vi "Analysis.SingleChannelLevelTransitionLogic.vi"(9 "Stimulus":dbl[](array[numeric]), 10 "Response":dbl[](array[numeric]), 11 "Parameters":T1) -> (3 "Fail":bool)   [LabVIEW 2014, in "NIAnalysis.lvlib"]
uses:
  NIAnalysis.lvlib
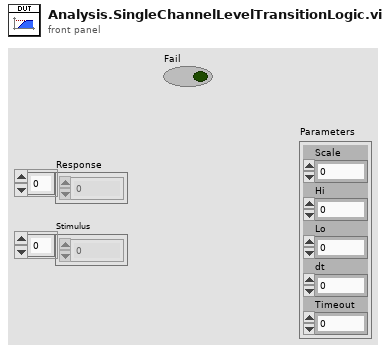
[diagram p1: front panel]
types:
  T1 = cluster{"Scale":dbl, "Hi":dbl, "Lo":dbl, "dt":dbl, "Timeout":dbl}
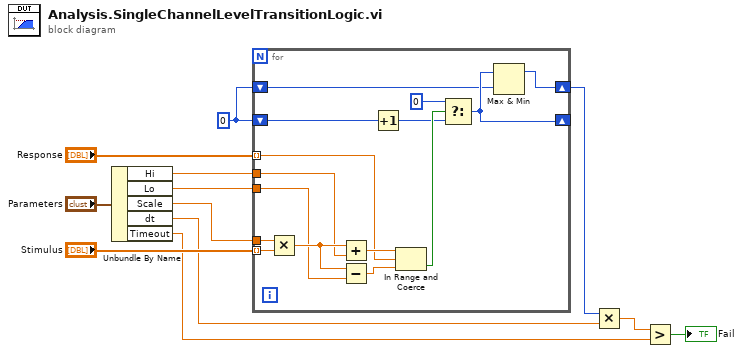
[diagram p0: block diagram]
diagram:
  w9 = u64 0
  n1 = Unbundle By Name("Parameters") -> ("Hi"=w4:dbl, "Lo"=w3:dbl, "Scale"=w5:dbl, "dt"=w2:dbl, "Timeout"=w1:dbl)
  n2 = for {
    tunnel: "Response" -> [w24] mode=indexing
    tunnel: "Stimulus" -> [w27] mode=indexing
    shift-right: [w19] -> _
    shift-left: w9 -> [w21]
    shift-right: [w18] -> w10
    shift-left: w9 -> [w17]
    tunnel: w5 -> [w15]
    tunnel: w4 -> [w14]
    tunnel: w3 -> [w13]
    n3 = Multiply(x=w15, y=w27) -> (x*y=w16:dbl)
    n4 = Add(x=w16, y=w14) -> (x+y=w26:dbl)
    n5 = Subtract(x=w16, y=w13) -> (x-y=w25:dbl)
    n6 = Increment(x=w21) -> (x+1=w20:u64)
    n7 = In Range and Coerce(upper limit=w26, x=w24, lower limit=w25) -> (In Range?=w23:bool)  [unwired: 1 out]
    n8 = Select(t=u64 0, s=w23, f=w20) -> (s? t:f=w19:u64)
    n9 = Max & Min(x=w19, y=w17) -> (max(x,y)=w18:u64)  [unwired: 1 out]
  }
  n10 = Multiply(x=w10, y=w2) -> (x*y=w11:dbl)
  n11 = Greater?(x=w11, y=w1) -> (0:→"Fail":bool)
